vi "p6.1 (hw7).vi"() -> (0 "Age (years)":i64)   [LabVIEW 2017]
doc: "Finds age in years of a person given the current date and the person's birth date as input."
panel:
  in  "Birth Date":T1
  in  "Current Date":T2
  # "Chapter 6 (P6.1)"
  # "Put in the Current date"
  # "Displays your age"
  # "Put in your Birth date"
  # "Patrik Sokolowski"
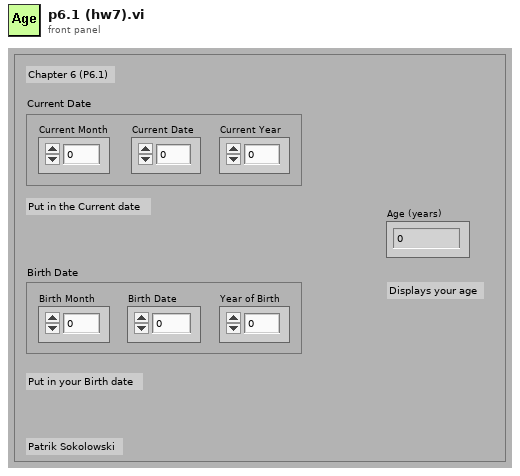
[diagram p1: front panel]
types:
  T1 = cluster{"Year of Birth":i64, "Birth Date":i64, "Birth Month":i64}
  T2 = cluster{"Current Year":i64, "Current Date":i64, "Current Month":i64}
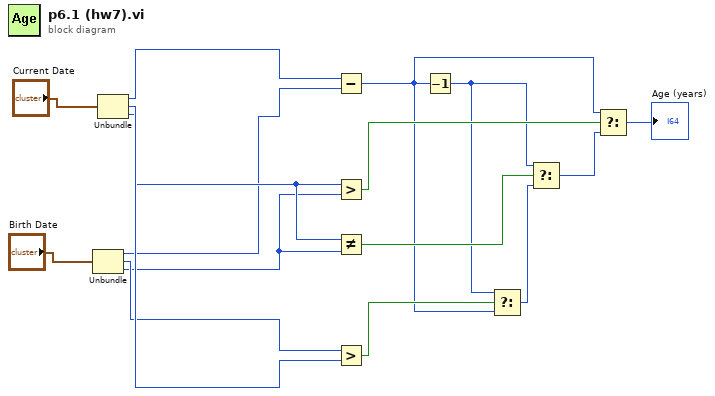
[diagram p0: block diagram]
diagram:
  n1 = Unbundle("Birth Date") -> ("Year of Birth"=w3:i64, "Birth Date"=w2:i64, "Birth Month"=w1:i64)
  n2 = Unbundle("Current Date") -> ("Current Year"=w7:i64, "Current Date"=w6:i64, "Current Month"=w5:i64)
  n3 = Subtract(x=w7, y=w3) -> (x-y=w9:i64)
  n4 = Greater?(x=w5, y=w1) -> (0:w15:bool)
  n5 = Not Equal?(x=w5, y=w1) -> (x != y?=w13:bool)
  n6 = Greater?(x=w2, y=w6) -> (0:w16:bool)
  n7 = Decrement(x=w9) -> (x-1=w10:i64)
  n8 = Select(t=w10, s=w16, f=w9) -> (s? t:f=w12:i64)
  n9 = Select(t=w10, s=w13, f=w12) -> (s? t:f=w14:i64)
  n10 = Select(t=w9, s=w15, f=w14) -> (s? t:f=→"Age (years)":i64)
